vi "Encase in Quotes.vi"(11 "String in":string) -> (3 "String out":string)   [LabVIEW 2014, in "C Header Generator.lvlib"]
uses:
  C Header Generator.lvlib
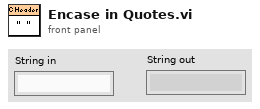
[diagram p1: front panel]
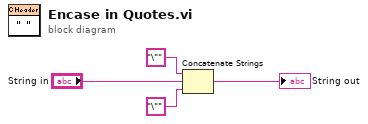
[diagram p0: block diagram]
diagram:
  n1 = Concatenate Strings("\"", "String in", "\"") -> (→"String out":string)
